vi "LoadOnly.vi"(8 "error in (no error)":errorcluster, 11 "Preferences in":refnum<class "SetListPrefs.lvclass">) -> (0 "error out":errorcluster, 2 "Raw XML":string, 3 "Preferences out":refnum<class "SetListPrefs.lvclass">)   [LabVIEW 2013, in "SetListPrefs.lvclass"]
uses:
  SetListPrefs.lvclass
  <vilib>/Utility/error.llb/DialogType.ctl
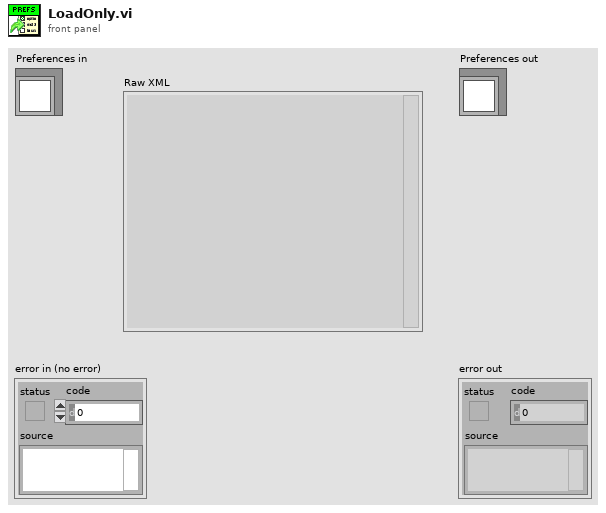
[diagram p1: front panel]
types:
  T1 = typedef "DialogType.ctl" = u16
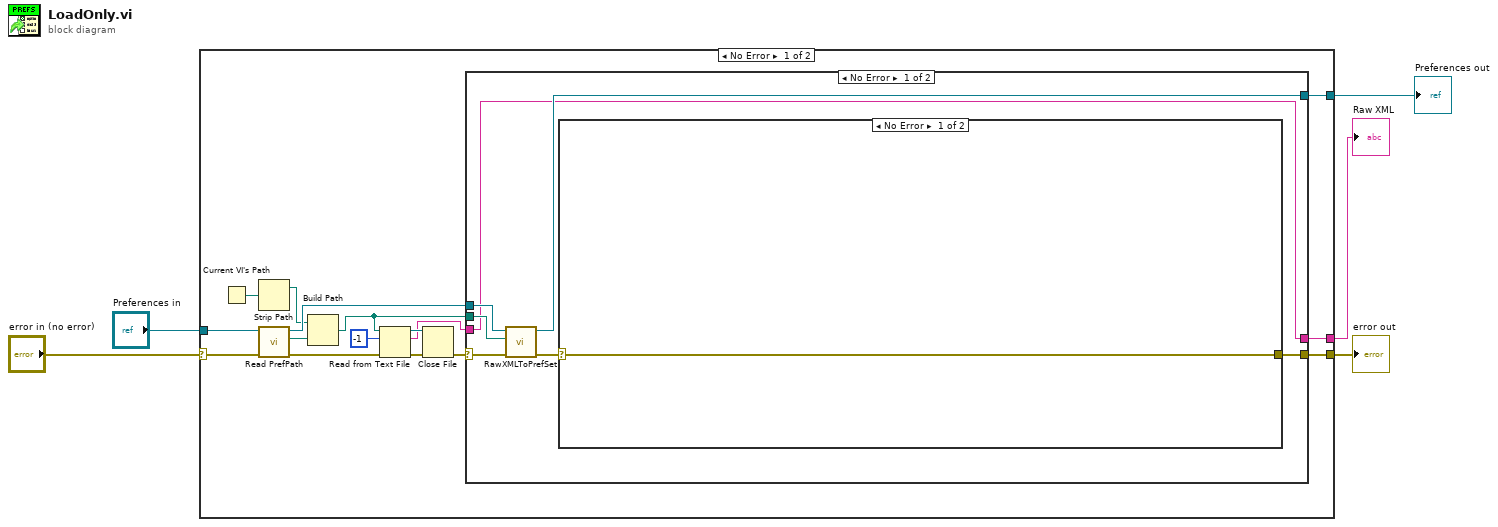
[diagram p0: block diagram]
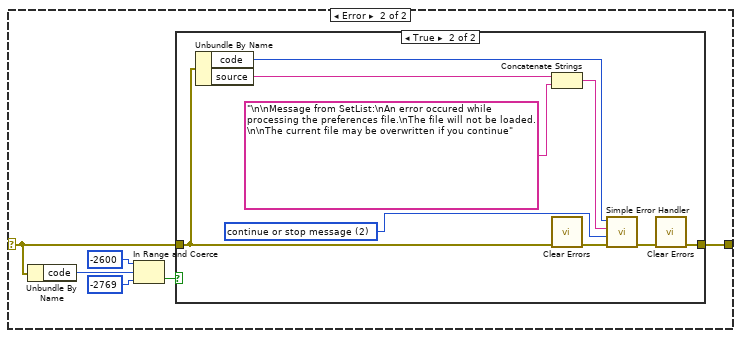
[diagram p2: hidden frame]
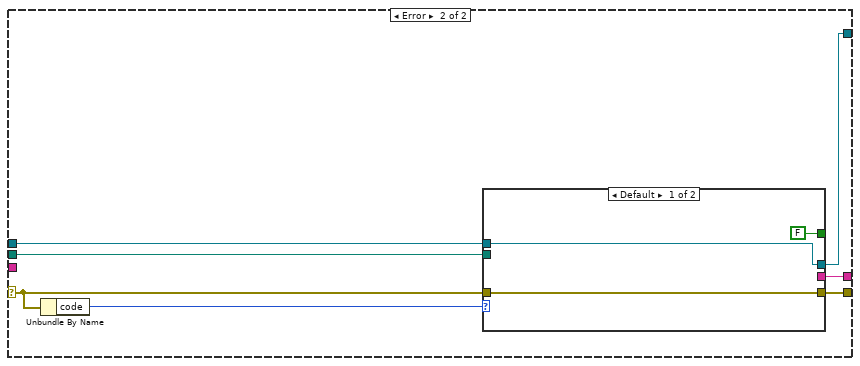
[diagram p4: hidden frame]
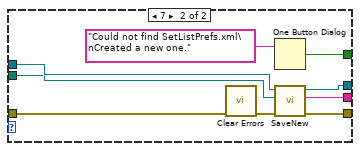
[diagram p5: hidden frame]
diagram:
  n1 = case shown="No Error" "error in (no error)" {
    selector: "error in (no error)" -> [w21 w66]
    tunnel: [w12 w66] -> w4
    tunnel: [w14 w65] -> w3
    tunnel: "Preferences in" -> [w20 w65]
    tunnel: [w8 _] -> w1
    frame No Error {
      n2 = Current VI's Path() -> (path=w7:path)
      n3 = Strip Path(path=w7) -> (stripped path=w6:path)  [unwired: 1 out]
      n4 = call-dynamic "Read PrefPath.vi"("error in (no error)"=w21, "Preferences in"=w20) -> ("error out"=w16:errorcluster, "PrefPath"=w19:path, "Preferences out"=w15:refnum<class "SetListPrefs.lvclass">)  [unwired: 7 in]
      n5 = Build Path(base path=w6, name or relative path=w19) -> (appended path=w11:path)
      n6 = Read from Text File(file (use dialog)=w11, count=-1, error in=w16) -> (refnum out=w17:refnum<file>, text=w9:string, error out=w18:errorcluster)  [unwired: 1 in, 1 out]
      n7 = Close File(refnum=w17, error in=w18) -> (error out=w13:errorcluster)  [unwired: 1 out]
      n8 = case shown="No Error" w13 {
        selector: w13 -> [w26 w46]
        tunnel: w15 -> [w28 w50]
        tunnel: [w27 w49] -> w14
        tunnel: [w22 w51] -> w12
        tunnel: [w24 w47] -> w8
        tunnel: w11 -> [w25 w48]
        tunnel: w9 -> [w24 _]
        frame No Error {
          n9 = call "RawXMLToPrefSet.vi"("error in (no error)"=w26, "path to XML document"=w25, "Preferences in"=w28) -> ("error out"=w23:errorcluster, "Preferences out"=w27:refnum<class "SetListPrefs.lvclass">)  [unwired: 7 in]
          n10 = case shown="No Error" w23 {
            selector: w23 -> [w29 w34]
            tunnel: [w29 w35] -> w22
            frame No Error {
            }
            frame Error {
              n11 = Unbundle By Name(w34) -> ("code"=w33:i32)
              n12 = In Range and Coerce(upper limit=-2600, x=w33, lower limit=-2769) -> (In Range?=w30:bool)  [unwired: 1 out]
              n13 = case shown="True" w30 {
                tunnel: w34 -> [w36 w41]
                tunnel: [w36 w44] -> w35
                frame False {
                }
                frame True {
                  w37 = T1 2 items=["no dialog", "OK message", "continue or stop message", "OK message + warnings", "continue/stop + warnings"] ("type of dialog (OK msg:1)")
                  n14 = Unbundle By Name(w41) -> ("code"=w43:i32, "source"=w38:string)
                  n15 = Concatenate Strings(w38, "\n\nMessage from SetList:\nAn error occured while processing the preferences file.\nThe file will not be loaded.\n\nThe current file may be overwritten if you continue" ("string")) -> (w42:string)
                  n16 = call <vilib>:"Clear Errors.vi"("error in (no error)"=w41) -> ("error out"=w40:errorcluster)  [unwired: 6 in]
                  n17 = call <vilib>:"Simple Error Handler.vi"("error code (no error:0)"=w43, "error source (\" \")"=w42, "type of dialog (OK msg:1)"=w37, "error in (no error)"=w40) -> ("error out"=w45:errorcluster)  [unwired: 1 in, 4 out]
                  n18 = call <vilib>:"Clear Errors.vi"("error in (no error)"=w45) -> ("error out"=w44:errorcluster)  [unwired: 6 in]
                }
              }
            }
          }
        }
        frame Error {
          n19 = Unbundle By Name(w46) -> ("code"=w52:i32)
          n20 = case shown="Default" w52 {
            tunnel: w46 -> [w55 w61]
            tunnel: [w55 w58] -> w51
            tunnel: w50 -> [w54 w64]
            tunnel: [w54 w63] -> w49
            tunnel: w48 -> [_ w60]
            tunnel: [_ w59] -> w47
            tunnel: [FALSE ("true") w57] -> _
            frame Default {
            }
            frame 7 {
              n21 = call <vilib>:"Clear Errors.vi"("error in (no error)"=w61) -> ("error out"=w62:errorcluster)  [unwired: 6 in]
              n22 = One Button Dialog(message="Could not find SetListPrefs.xml\nCreated a new one.") -> (true=w57:bool)  [unwired: 1 in]
              n23 = call "SaveNew.vi"("error in (no error)"=w62, "Path"=w60, "Preferences in"=w64) -> ("error out"=w58:errorcluster, "Raw XML"=w59:string, "Preferences out"=w63:refnum<class "SetListPrefs.lvclass">)  [unwired: 6 in]
            }
          }
        }
      }
    }
    frame Error {
    }
  }
  "error out" <- w4
  "Preferences out" <- w3
  "Raw XML" <- w1
